vi "Select Phase-Lock Mode.vi"(8 "error in (no error)":errorcluster, 10 "Mode (1:Phase-Locked)":i32(ring)=1 items=["Phase-Locked"=1, "Independent"=2], 11 "VISA resource name":refnum<visa-resource-name>) -> (0 "error out":errorcluster, 3 "VISA resource name out":refnum<visa-resource-name>)   [LabVIEW 2017, in "Siglent SDG 1000 5000 800 Series.lvlib"]
doc: "Enables or disables the output of the selected channel."
uses:
  <instrlib>/Siglent SDG 1000 5000 800 Series/Siglent SDG 1000 5000 800 Series.lvlib
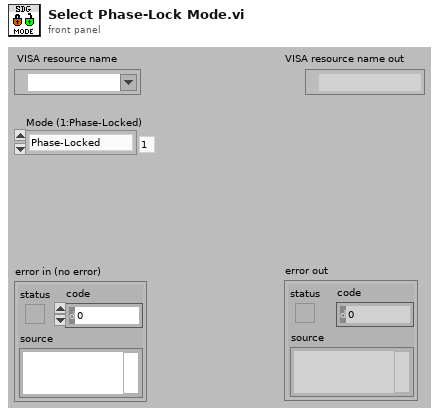
[diagram p1: front panel]
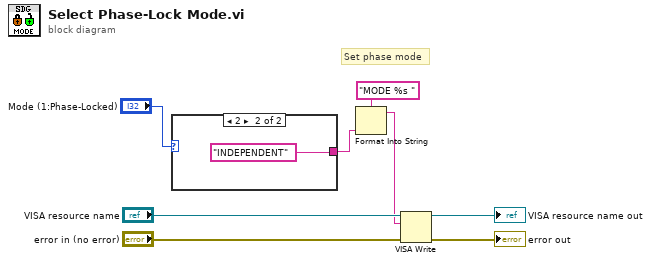
[diagram p0: block diagram]
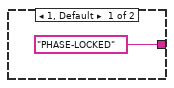
[diagram p2: hidden frame]
diagram:
  # "Set phase mode"
  n1 = case shown="2" "Mode (1:Phase-Locked)" {
    tunnel: ["PHASE-LOCKED" ("input 1") "INDEPENDENT" ("input 1")] -> w1
    frame 1, Default {
    }
    frame 2 {
    }
  }
  n2 = Format Into String(format string="MODE %s ", w1) -> (resulting string=w3:string)  [unwired: 2 in, 1 out]
  n3 = VISA Write(VISA resource name="VISA resource name", write buffer=w3, error in (no error)="error in (no error)") -> (VISA resource name out=→"VISA resource name out":refnum<visa-resource-name>, error out=→"error out":errorcluster)  [unwired: 1 out]
